vi "Construct ModelSubscribesToDoubleFloatX.vi"() -> (1 "Test Result Notifier":refnum<notifier>, 3 "ModelSubscribesToDoubleFloatX":refnum<class "ModelSubscribesToDoubleFloatX.lvclass">)   [LabVIEW 2017, in "ModelSubscribesToDoubleFloatX.lvclass"]
uses:
  ModelSubscribesToDoubleFloatX.lvclass
  ModelSubscribesToDoubleFloatX.lvclass/ModelSubscribesToDoubleFloatX.ctl
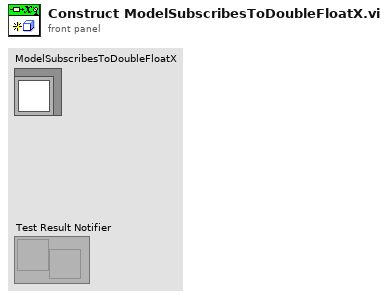
[diagram p1: front panel]
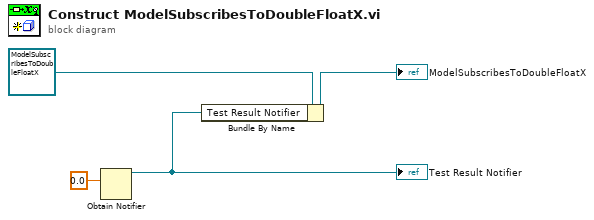
[diagram p0: block diagram]
diagram:
  n1 = Obtain Notifier(notification data type=0.0) -> (notifier out=w1:refnum<notifier>)  [unwired: 3 in, 2 out]
  "Test Result Notifier" <- w1
  n2 = Bundle By Name(cluster=refnum<class "ModelSubscribesToDoubleFloatX.lvclass"> refnum ("ModelSubscribesToDoubleFloatX in"), "Test Result Notifier"=w1) -> (→"ModelSubscribesToDoubleFloatX":refnum<class "ModelSubscribesToDoubleFloatX.lvclass">)
